vi "Risk Weight.vi"(10 "Accident Position":T1[](array[typedef]), 11 "Map":i32[][](array[numeric])) -> (3 "Map Out":i32[][](array[numeric]))   [LabVIEW 2015]
uses:
  Data Def/Accident Position.ctl
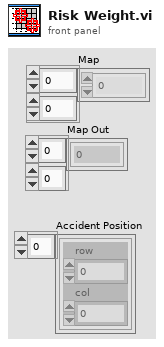
[diagram p1: front panel]
types:
  T1 = typedef "Accident Position.ctl" = cluster{"row":i32, "col":i32}
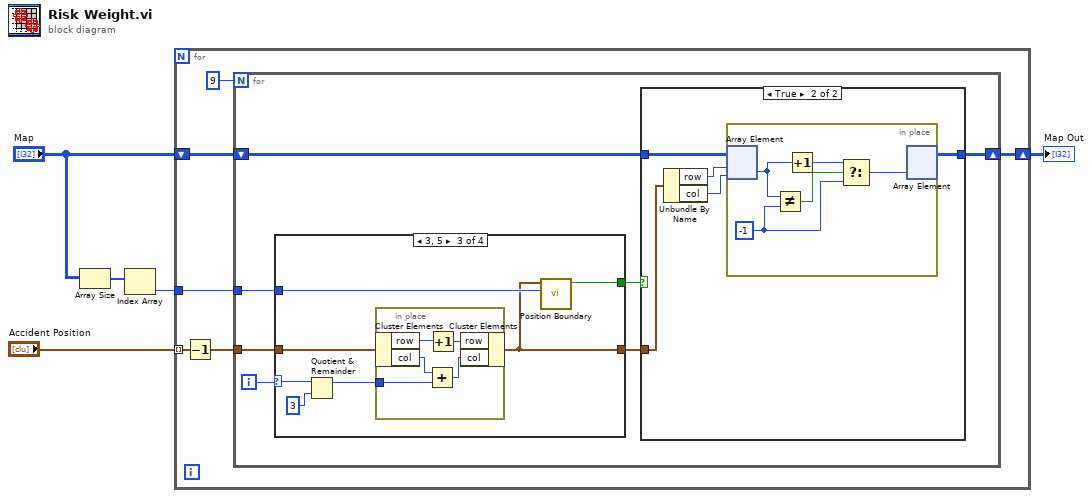
[diagram p0: block diagram]
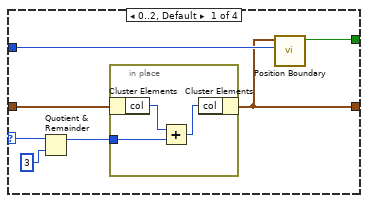
[diagram p3: hidden frame]
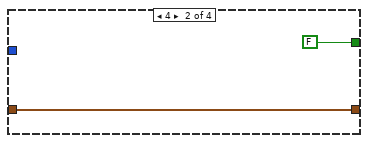
[diagram p4: hidden frame]
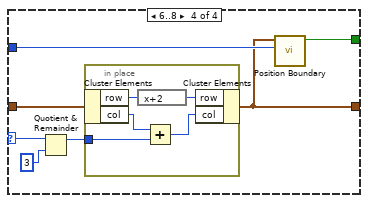
[diagram p5: hidden frame]
diagram:
  n1 = Array Size(array="Map") -> (size(s)=w4:i32[])
  n2 = Index Array(array=w4) -> (element=w3:i32)  [unwired: 1 in]
  n3 = for {
    tunnel: "Accident Position" -> [w8] mode=indexing
    tunnel: w3 -> [w10]
    shift-right: [w6] -> w1
    shift-left: "Map" -> [w7]
    n4 = Decrement(x=w8) -> (x-1=w9:T1)
    n5 = for {
      N: 9 -> [_]
      tunnel: w9 -> [w18]
      tunnel: w10 -> [w17]
      shift-right: [w12] -> w6
      shift-left: w7 -> [w14]
      i -> [w16]
      n6 = case shown="3, 5" w16 {
        selector: w16 -> [w32 _ w44 w56]
        tunnel: w18 -> [w34 w40 w46 w58]
        tunnel: [w33 w40 w45 w57] -> w13
        tunnel: w17 -> [w36 _ w48 w60]
        tunnel: [w35 FALSE ("In Range?") w47 w59] -> w15
        frame 0..2, Default {
          n7 = Quotient & Remainder(x=w32, y=3) -> (x-y*floor(x/y)=w30:i32)  [unwired: 1 out]
          n8 = in-place {
            in-place-border: w30 -> [w38]
            n9 = in-place-cluster #1(w34) -> ("col"=w39:i32)
            n10 = Add(x=w39, y=w38) -> (x+y=w37:i32)
            n11 = in-place-cluster #1("col"=w37) -> (w33:T1)
          }
          n12 = call "Position Boundary.vi"("NxN"=w36, "Accident Position"=w33) -> ("In Range?"=w35:bool)  [unwired: 9 in]
        }
        frame 4 {
        }
        frame 3, 5 {
          n13 = Quotient & Remainder(x=w44, y=3) -> (x-y*floor(x/y)=w42:i32)  [unwired: 1 out]
          n14 = in-place {
            in-place-border: w42 -> [w52]
            n15 = in-place-cluster #2(w46) -> ("row"=w50:i32, "col"=w53:i32)
            n16 = Add(x=w53, y=w52) -> (x+y=w51:i32)
            n17 = Increment(x=w50) -> (x+1=w49:i32)
            n18 = in-place-cluster #2("row"=w49, "col"=w51) -> (w45:T1)
          }
          n19 = call "Position Boundary.vi"("NxN"=w48, "Accident Position"=w45) -> ("In Range?"=w47:bool)  [unwired: 9 in]
        }
        frame 6..8 {
          n20 = Quotient & Remainder(x=w56, y=3) -> (x-y*floor(x/y)=w54:i32)  [unwired: 1 out]
          n21 = in-place {
            in-place-border: w54 -> [w64]
            n22 = in-place-cluster #3(w58) -> ("row"=w62:i32, "col"=w65:i32)
            n23 = expression code="x+2"(w62) -> (w61:i32)
            n24 = Add(x=w65, y=w64) -> (x+y=w63:i32)
            n25 = in-place-cluster #3("row"=w61, "col"=w63) -> (w57:T1)
          }
          n26 = call "Position Boundary.vi"("NxN"=w60, "Accident Position"=w57) -> ("In Range?"=w59:bool)  [unwired: 9 in]
        }
      }
      n27 = case shown="True" w15 {
        tunnel: w14 -> [w19 w24]
        tunnel: w13 -> [_ w23]
        tunnel: [w19 w20] -> w12
        frame False {
        }
        frame True {
          n28 = Unbundle By Name(w23) -> ("row"=w22:i32, "col"=w21:i32)
          n29 = in-place {
            w28 = -1 ("y")
            n30 = in-place-array #4(w24, w22, w21) -> (w27:i32)
            n31 = Not Equal?(x=w27, y=w28) -> (x != y?=w29:bool)
            n32 = Increment(x=w27) -> (x+1=w25:i32)
            n33 = Select(t=w25, s=w29, f=w28) -> (s? t:f=w26:i32)
            n34 = in-place-array #4(w26) -> (w20:i32[][])  [unwired: 2 out]
          }
        }
      }
    }
  }
  "Map Out" <- w1
